vi "Testbench.vi"() -> ()   [LabVIEW 2015]
doc: "123456"
uses:
  <vilib>/ActorFramework/Actor/Actor.lvclass
  Model/Model.lvclass
  <vilib>/ActorFramework/Stop Msg/Stop Msg.lvclass
  Model Messages/Load Project from Path Msg/Load Project from Path Msg.lvclass
  Model Messages/Load Project from Reference Msg/Load Project from Reference Msg.lvclass
  Model Messages/Add VI from File Msg/Add VI from File Msg.lvclass
panel:
  in  "Add VI from File":bool
  in  "VI Path":path
  in  "Ring":u16(ring) items=["Actor Documentation Tool.lvproj"]
  in  "Open Project In Memory":bool
  in  "Path":path
  in  "Open Project From File":bool
  in  "Stop":bool
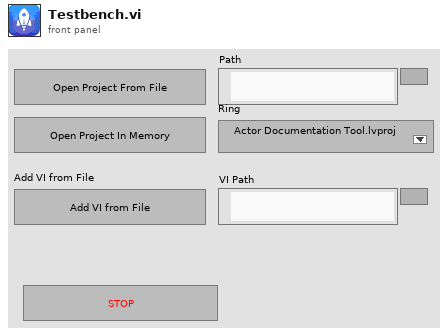
[diagram p1: front panel]
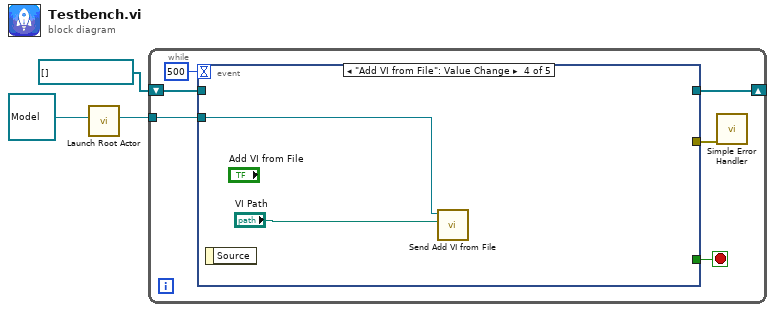
[diagram p0: block diagram]
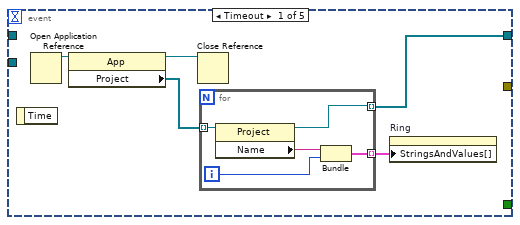
[diagram p2: hidden frame]
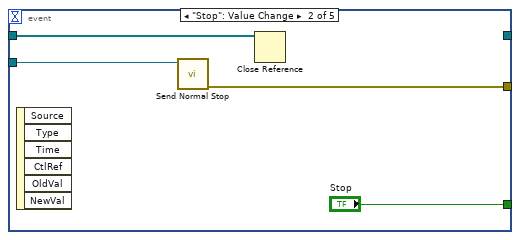
[diagram p3: hidden frame]
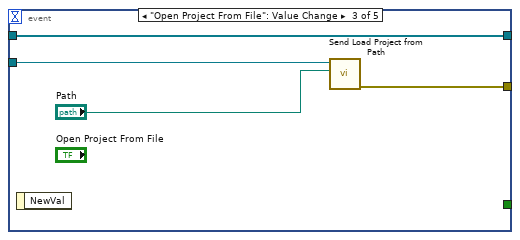
[diagram p4: hidden frame]
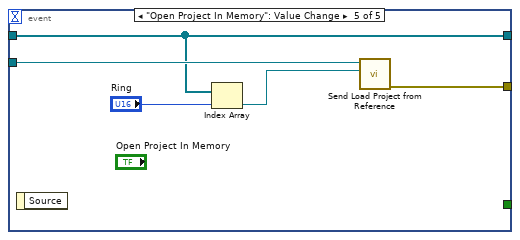
[diagram p5: hidden frame]
diagram:
  n1 = call <vilib>:"Launch Root Actor.vi"("Actor"=refnum<class "Model.lvclass"> refnum ("Model.lvlib:Model.lvclass")) -> ("Actor's Enqueuer"=w2:refnum<class "Message Enqueuer.lvclass">)  [unwired: 9 in, 1 out]
  n2 = while {
    tunnel: w2 -> [w9]
    shift-right: [w5] -> _
    shift-left: refnum<vi>[] [] -> [w4]
    stop <- w8 stop-if-true
    n3 = event shown="[3] \"Add VI from File\": Value Change" {
      selector: _ -> [_ _ _ _ _]
      dyn-events: _ -> [_ _ _ _ _]
      timeout: 500 -> [_ _ _ _ _]
      tunnel: w9 -> [_ w23 w27 w29 w34]
      tunnel: [_ "Stop" _ _ _] -> w8
      tunnel: [_ w21 w26 _ w33] -> w7
      tunnel: [w11 _ w24 _ w32] -> w5
      tunnel: w4 -> [_ w20 w24 _ w32]
      event Timeout {
        n4 = event-data() -> ()  [unwired: 1 in, 1 out]
        n5 = Open Application Reference() -> (3:w13:refnum<vi>)  [unwired: 4 in, 1 out]
        n6 = property class="App"(reference=w13) -> (reference out=w12:refnum<vi>, "Project"=w14:refnum<vi>[])  [unwired: 1 in, 1 out]
        n7 = Close Reference(reference=w12) -> ()  [unwired: 1 in, 1 out]
        n8 = for {
          tunnel: w14 -> [w19] mode=indexing
          tunnel: [w18] -> w11 mode=indexing
          tunnel: [w15] -> w10 mode=indexing
          i -> [w16]
          n9 = property class="Project"(reference=w19) -> (reference out=w18:refnum<vi>, "Name"=w17:string)  [unwired: 1 in, 1 out]
          n10 = Bundle("Name"=w17, w16) -> (w15:cluster{"Name":string, i32})  [unwired: 1 in]
        }
        n11 = property on="Ring" class="Ring (strict)"("StringsAndValues[]"=w10) -> ()  [unwired: 2 in, 2 out]
      }
      event "Stop": Value Change {
        n12 = event-data() -> ()  [unwired: 1 in, 6 out]
        n13 = call <vilib>:"Send Normal Stop.vi"("Message Enqueuer"=w23) -> ("error out"=w21:errorcluster)  [unwired: 10 in]
        n14 = Close Reference(reference=w20) -> ()  [unwired: 1 in, 1 out]
      }
      event "Open Project From File": Value Change {
        n15 = event-data() -> ()  [unwired: 1 in, 1 out]
        n16 = call "Send Load Project from Path.vi"("Project Path"="Path", "Message Enqueuer"=w27) -> ("error out"=w26:errorcluster)  [unwired: 8 in, 1 out]
      }
      event "Add VI from File": Value Change {
        n17 = event-data() -> ()  [unwired: 1 in, 1 out]
        n18 = call "Send Add VI from File.vi"("VI Path"="VI Path", "Message Enqueuer"=w29) -> ()  [unwired: 8 in, 2 out]
      }
      event "Open Project In Memory": Value Change {
        n19 = event-data() -> ()  [unwired: 1 in, 1 out]
        n20 = Index Array(array=w32, index="Ring") -> (element=w31:refnum<vi>)
        n21 = call "Send Load Project from Reference.vi"("Project Reference"=w31, "Message Enqueuer"=w34) -> ("error out"=w33:errorcluster)  [unwired: 8 in, 1 out]
      }
    }
    n22 = call <vilib>:"Simple Error Handler.vi"("error in (no error)"=w7) -> ()  [unwired: 4 in, 5 out]
  }
